vi "GenerateTestImage.vi"(0 "spotsize":sgl=20.0, 4 "ypos":sgl=128.0, 5 "height":u32=256, 6 "xpos":sgl=128.0, 7 "image":T1, 8 "maxphotoncount":sgl, 9 "width":u32=256) -> (2 "Image":T1(plugin-control))   [LabVIEW 2011]
uses:
  <vilib>/vision/Image Controls.llb/IMAQ Image.ctl
  TrackerDLL.vi
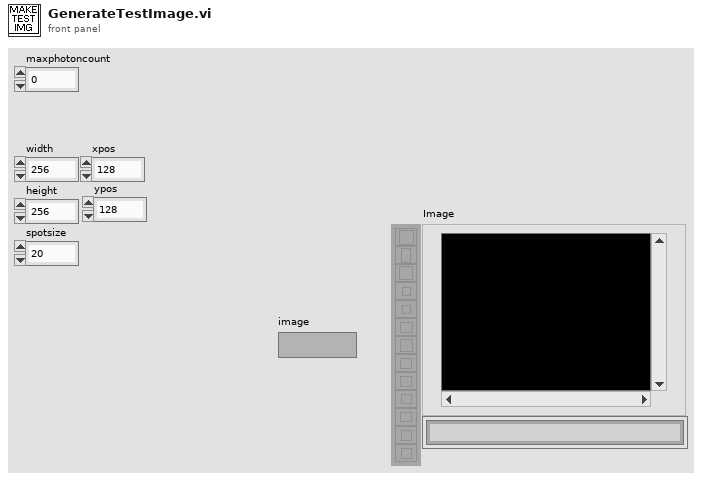
[diagram p1: front panel]
types:
  T1 = typedef "IMAQ Image.ctl" = refnum<image>
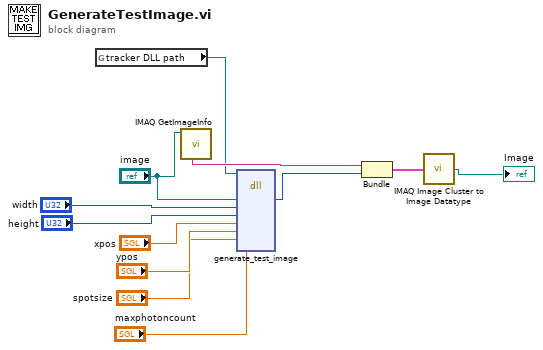
[diagram p0: block diagram]
diagram:
  n1 = global read "TrackerDLL.vi" "tracker DLL path"() -> (w2:path)
  n2 = call "IMAQ GetImageInfo"("Image"="image") -> ("Image Name"=w6:string)  [unwired: 3 in, 7 out]
  n3 = dll-call lib="D:/jcnossen1/cudaqi-tracker/cputrack/cputrack_d.dll" fn="generate_test_image"(path in=w2, "image"="image", "width"="width", "height"="height", "xpos"="xpos", "ypos"="ypos", "spotsize"="spotsize", "maxphotoncount"="maxphotoncount") -> ("image"=w4:u64)  [unwired: 9 in, 2 out]
  n4 = Bundle("Image Name"=w6, "image"=w4) -> (w7:cluster{"Image Name":string, "image":u64})  [unwired: 1 in]
  n5 = call <vilib>:"IMAQ Image Cluster to Image Datatype.vi"("Image"=w7) -> ("Image (dup)"=→"Image":T1)
